vi "VISA_Write+Read.vi"(7 "Read?(T)":bool=TRUE, 8 "error in (no error)":errorcluster, 10 "Write Buffer":string, 11 "VISA resource name":refnum<visa-resource-name>) -> (0 "error out":errorcluster, 2 "readout":string, 3 "VISA resource name out":refnum<visa-resource-name>)   [LabVIEW 2012, in "ESP300.lvlib"]
doc: "This Utility VI is a wrapper which writes to the instrument and reads the response. This VI is intended to be used as a private VI and altering it could cause several public VI's to operate incorrectly."
uses:
  ESP300.lvlib
  <vilib>/Utility/error.llb/DialogType.ctl
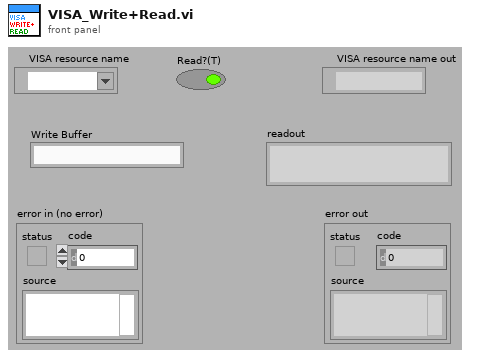
[diagram p1: front panel]
types:
  T1 = typedef "DialogType.ctl" = u16
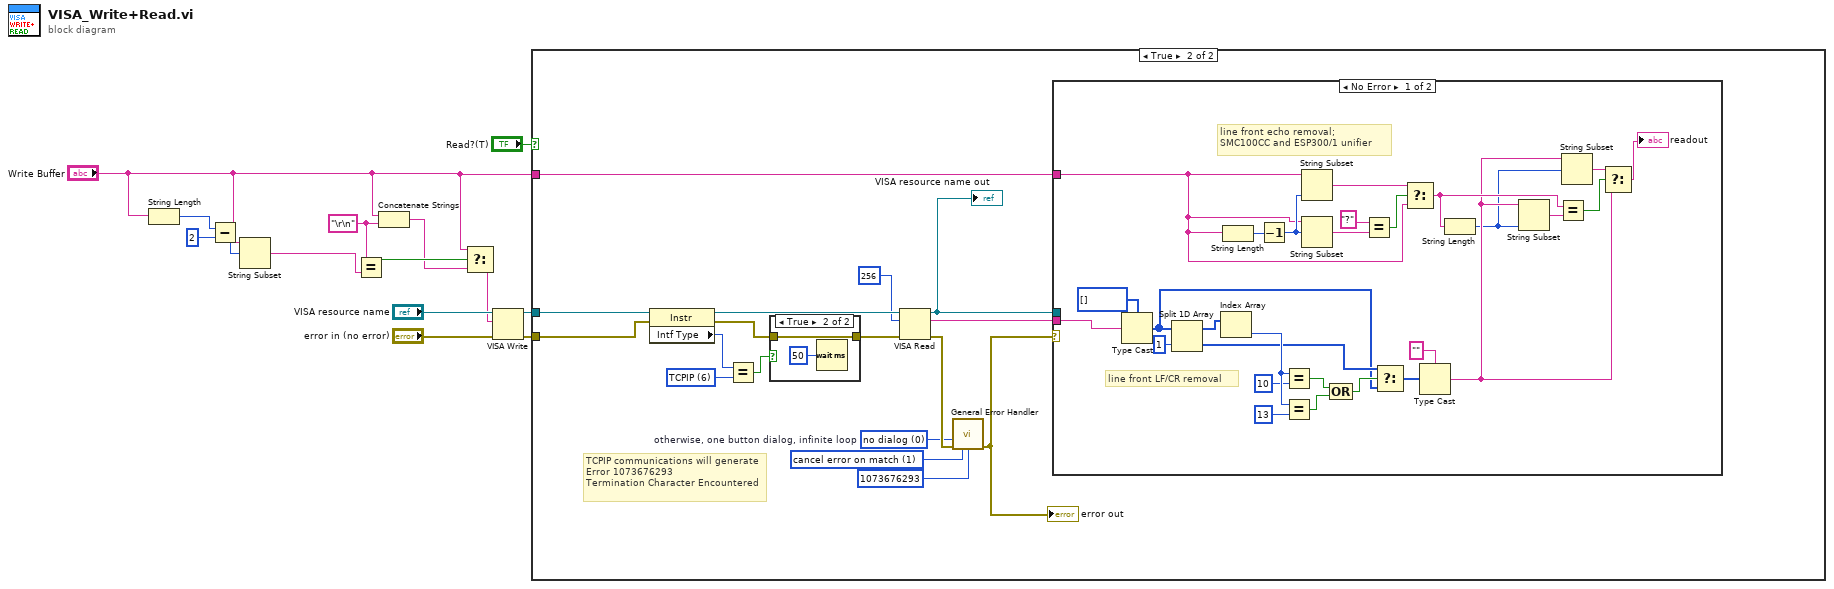
[diagram p0: block diagram]
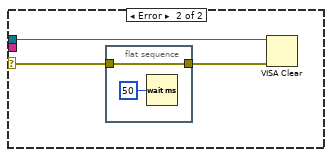
[diagram p3: hidden frame]
diagram:
  w4 = "\r\n"
  n1 = String Length(string="Write Buffer") -> (length=w8:i32)
  n2 = Subtract(x=w8, y=2) -> (x-y=w6:i32)
  n3 = String Subset(string="Write Buffer", offset (0)=w6) -> (substring=w3:string)  [unwired: 1 in]
  n4 = Equal?(x=w4, y=w3) -> (x = y?=w5:bool)
  n5 = Concatenate Strings("Write Buffer", w4) -> (w1:string)
  n6 = Select(t="Write Buffer", s=w5, f=w1) -> (s? t:f=w9:string)
  n7 = VISA Write(VISA resource name="VISA resource name", write buffer=w9, error in (no error)="error in (no error)") -> (VISA resource name out=w12:refnum<visa-resource-name>, error out=w11:errorcluster)  [unwired: 1 out]
  n8 = case shown="True" "Read?(T)" {
    tunnel: w12 -> [_ w26]
    tunnel: w11 -> [_ w20]
    tunnel: "Write Buffer" -> [_ w18]
    frame False {
    }
    frame True {
      w17 = T1 0 items=["no dialog", "OK message", "continue or stop message", "OK message + warnings", "continue/stop + warnings"]  # otherwise, one button dialog, infinite loop
      w23 = u16 6 items=["GPIB"=1, "VXI"=2, "GPIB-VXI"=3, "Serial"=4, "PXI"=5, "TCPIP"=6, "USB"=7, "FireWire"=9] ("Interface Information:Interface Type")
      w31 = 1 items=["no exception", "cancel error on match", "set error on match"] ("[exception action] (none:0)")
      # "TCPIP communications will generate\nError 1073676293\nTermination Character Encountered"
      n9 = property class="Instr"(reference=w26, error in=w20) -> (reference out=w25:refnum<visa-resource-name>, error out=w27:errorcluster, "Intf Type"=w22:u16)
      n10 = Equal?(x=w22, y=w23) -> (x = y?=w24:bool)
      n11 = case shown="True" w24 {
        tunnel: [w65 w66] -> w28
        tunnel: w27 -> [w65 w66]
        frame False {
        }
        frame True {
          n12 = Wait (ms)(milliseconds to wait=u32 50) -> ()  [unwired: 1 out]
        }
      }
      n13 = VISA Read(VISA resource name=w25, byte count=u32 256, error in (no error)=w28) -> (VISA resource name out=w15:refnum<visa-resource-name>, read buffer=w19:string, error out=w29:errorcluster)  [unwired: 1 out]
      "VISA resource name out" <- w15
      n14 = call <vilib>:"General Error Handler.vi"("type of dialog (OK msg:1)"=w17, "error in (no error)"=w29, "[exception action] (none:0)"=w31, "[exception code]"=1073676293) -> ("error out"=w16:errorcluster)  [unwired: 7 in, 4 out]
      "error out" <- w16
      n15 = case shown="No Error" w16 {
        selector: w16 -> [_ w60]
        tunnel: w19 -> [w34 _]
        tunnel: w18 -> [w33 _]
        tunnel: w15 -> [_ w62]
        frame No Error {
          # "line front LF/CR removal"
          # "line front echo removal;\nSMC100CC and ESP300/1 unifier"
          n16 = Type Cast(type=u8[] [], x=w34) -> (*(type *) &x=w49:u8[])
          n17 = Split 1D Array(array=w49, index=1) -> (first subarray=w54:u8[], second subarray=w50:u8[])
          n18 = Index Array(array=w54) -> (element=w53:u8)  [unwired: 1 in]
          n19 = String Length(string=w33) -> (length=w43:i32)
          n20 = Decrement(x=w43) -> (x-1=w36:i32)
          n21 = Equal?(x=w53, y=u8 10) -> (x = y?=w58:bool)
          n22 = Equal?(x=w53, y=u8 13) -> (x = y?=w59:bool)
          n23 = String Subset(string=w33, length (rest)=w36) -> (substring=w42:string)  [unwired: 1 in]
          n24 = String Subset(string=w33, offset (0)=w36) -> (substring=w46:string)  [unwired: 1 in]
          n25 = Compound Arithmetic op=OR(w58, w59) -> (w57:bool)
          n26 = Equal?(x="?" ("regular expression"), y=w46) -> (x = y?=w44:bool)
          n27 = Select(t=w50, s=w57, f=w49) -> (s? t:f=w48:u8[])
          n28 = Select(t=w42, s=w44, f=w33) -> (s? t:f=w40:string)
          n29 = Type Cast(type="" ("read buffer"), x=w48) -> (*(type *) &x=w37:string)
          n30 = String Length(string=w40) -> (length=w35:i32)
          n31 = String Subset(string=w37, length (rest)=w35) -> (substring=w41:string)  [unwired: 1 in]
          n32 = Equal?(x=w40, y=w41) -> (x = y?=w39:bool)
          n33 = String Subset(string=w37, offset (0)=w35) -> (substring=w38:string)  [unwired: 1 in]
          n34 = Select(t=w38, s=w39, f=w37) -> (s? t:f=→"readout":string)
        }
        frame Error {
          n35 = flat-sequence {
            tunnel: [w63] -> w61
            tunnel: w60 -> [w63]
            frame #0 {
              n36 = Wait (ms)(milliseconds to wait=u32 50) -> ()  [unwired: 1 out]
            }
          }
          n37 = VISA Clear(VISA resource name=w62, error in (no error)=w61) -> ()  [unwired: 2 out]
        }
      }
    }
  }
